vi "Create.vi"(8 "error in (no error)":errorcluster, 10 "value in":variant, 11 "User Defined in":refnum<class "User Defined.lvclass">) -> (0 "error out":errorcluster, 2 "value out":variant, 3 "User Defined out":refnum<class "User Defined.lvclass">)   [LabVIEW 2020, in "PV Access.lvlib" / "PV Data.lvlib" / "User Defined.lvclass"]
uses:
  User Defined.lvclass
  User Defined.lvclass/User Defined.ctl
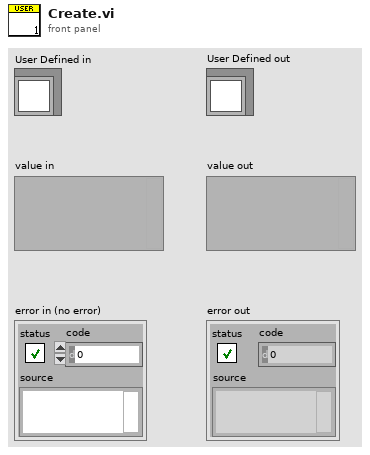
[diagram p1: front panel]
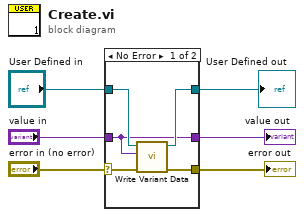
[diagram p0: block diagram]
diagram:
  n1 = case shown="No Error" "error in (no error)" {
    selector: "error in (no error)" -> [w11 w14]
    tunnel: [w10 w14] -> w5
    tunnel: [w7 w13] -> w3
    tunnel: "value in" -> [w7 w13]
    tunnel: [w9 w12] -> w2
    tunnel: "User Defined in" -> [w8 w12]
    frame No Error {
      n2 = call-dynamic "Write Variant Data.vi"("error in (no error)"=w11, "data"=w7, "Base in"=w8) -> ("error out"=w10:errorcluster, "Base out"=w9:refnum<class "User Defined.lvclass">)  [unwired: 7 in]
    }
    frame Error {
    }
  }
  "error out" <- w5
  "User Defined out" <- w2
  "value out" <- w3
